vi "Actor Core.vi"(8 "error in":errorcluster, 11 "POLARIS Target Focus Actor in":refnum<class "POLARIS Target Focus Actor.lvclass">) -> (0 "error out":errorcluster, 3 "Actor out":refnum<class "Actor.lvclass">)   [LabVIEW 2014, in "POLARIS Target Focus Actor.lvlib" / "POLARIS Target Focus Actor.lvclass"]
doc: "(<B>Filename</B>: Actor Framework.lvlib:Actor.lvclass:Actor Core.vi)\n\nReceives messages to the actor, reacts to them, and initiates any error handling that may shut the actor down.\n\nDescendant classes may override this VI to append parallel tasks for the actor to complete while it handles messages. Overrides use the Call Parent Method node."
uses:
  POLARIS Target Focus Actor.lvclass
  <vilib>/ActorFramework/Actor/Actor.lvclass
  Utility/Width Method.ctl
  POLARIS TA Focus Display/POLARIS TA Focus Display/POLARIS TA Focus Display.lvclass
  Analyze/Analyze Parameter/Analyze Parameter Energy/Analyze Parameter Energy.lvclass
  Analyze/Analyze Parameter/Analyze Parameter Width Method/Width Method.lvclass
  Analyze/Analyze Parameter/Analyze Parameter Fluence/Analyze Parameter Fluence.lvclass
  Analyze/Analyze Classes/Analyze Q-Factor/Analyze q-Factor.lvclass
  Analyze/Results and Overlays/Results q-Factor/Analyze Results q-Factor.lvclass
  Camera Actors/IMAQdx Actor/IMAQdx Actor/IMAQdx Actor.lvclass
  Display Actors/HIJ Vision Display/HIJ Vision Display/HIJ Vision Display.lvclass/HIJ Vision Display.ctl
  POLARIS Target Focus Actor.lvclass/POLARIS Target Focus Actor.ctl
  Analyze/Analyze Parameter/Analyze Parameter Energy/Analyze Parameter Energy.lvclass/Analyze Parameter Energy.ctl
  Analyze/Results and Overlays/Results q-Factor/Analyze Results q-Factor.lvclass/Analyze Results q-Factor.ctl
  Applications/HIJ Vision Application/HIJ Vision Application/HIJ Vision Application.lvclass/HIJ Vision Application.ctl
  Applications/HIJ Vision Camera App/HIJ Vision Camera App/HIJ Vision Camera App.lvclass/HIJ Vision Camera App.ctl
  Shared Code/Viewable Actor/ViewableActor/ViewableActor.lvclass/ViewableActor.ctl
  <vilib>/ActorFramework/Actor/Actor.lvclass/Actor.ctl
  <vilib>/ActorFramework/Message Enqueuer/Message Enqueuer.lvclass/Message Enqueuer.ctl
  Applications/HIJ Vision Application/HIJ Vision Application Messages/Set Parameter Msg/Set Parameter Msg.lvclass/Set Parameter Msg.ctl
  Analyze/Analyze Parameter/Analyze Parameter Energy/Write Energy.vi
  Analyze/Results and Overlays/Results q-Factor/Write A ref .vi
  Analyze/Results and Overlays/Results q-Factor/Write q ref.vi
  Display Actors/HIJ Vision Display/HIJ Vision Display/Write Save Report_.vi
  Applications/HIJ Vision Application/HIJ Vision Application/Write SubPnl for Display.vi
  Applications/HIJ Vision Camera App/HIJ Vision Camera App/Write Child Menu.vi
  Applications/HIJ Vision Application/HIJ Vision Application/Write HIJ Vision Display.vi
  Applications/HIJ Vision Application/HIJ Vision Application/Write Analyze Objs.vi
  Applications/HIJ Vision Camera App/HIJ Vision Camera App/Write Camera Actor.vi
  Shared Code/Viewable Actor/ViewableActor/Write UI VI Ref.vi
  <vilib>/ActorFramework/Message Enqueuer/Init from Existing Queue.vi
  <vilib>/ActorFramework/Message Enqueuer/Enqueue.vi
  <vilib>/ActorFramework/Message Priority Queue/Priority Enqueue.vi
  <vilib>/ActorFramework/Message Enqueuer/Message Enqueuer.lvclass
  <vilib>/ActorFramework/Stop Msg/Stop Msg.lvclass
  Applications/HIJ Vision Application/HIJ Vision Application Messages/Set Parameter Msg/Set Parameter Msg.lvclass
  Applications/HIJ Vision Camera App/HIJ Vision Camera App/HIJ Vision Camera App.lvclass
  Utility/POLARIS Vision utility.lvlib
panel:
  in  "Stop Signal":bool
  out "q-Factor":dbl format="%#_3g"
  out "A":dbl[unit] format="%#.1g"
  out "I [W/cm^2]":dbl[unit] format="%#.2g"
  in  "Energy":dbl[unit]=10.0
  in  "Size of hot Region":i32=10
  in  "Method":T1
  in  "Pulse duration":dbl[unit]=1e-13
  in  "Compressor eff.":dbl=0.63
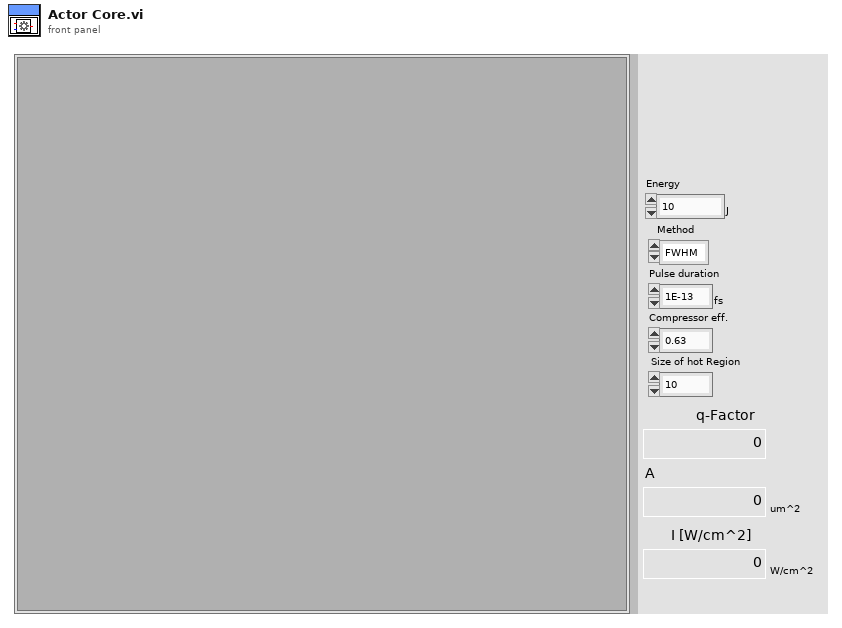
[diagram p1: front panel]
types:
  T1 = typedef "POLARIS Vision utility.lvlib/Width Method.ctl" = enum16{"FWHM", "1/e", "1/e^2", "80%", "90%"}
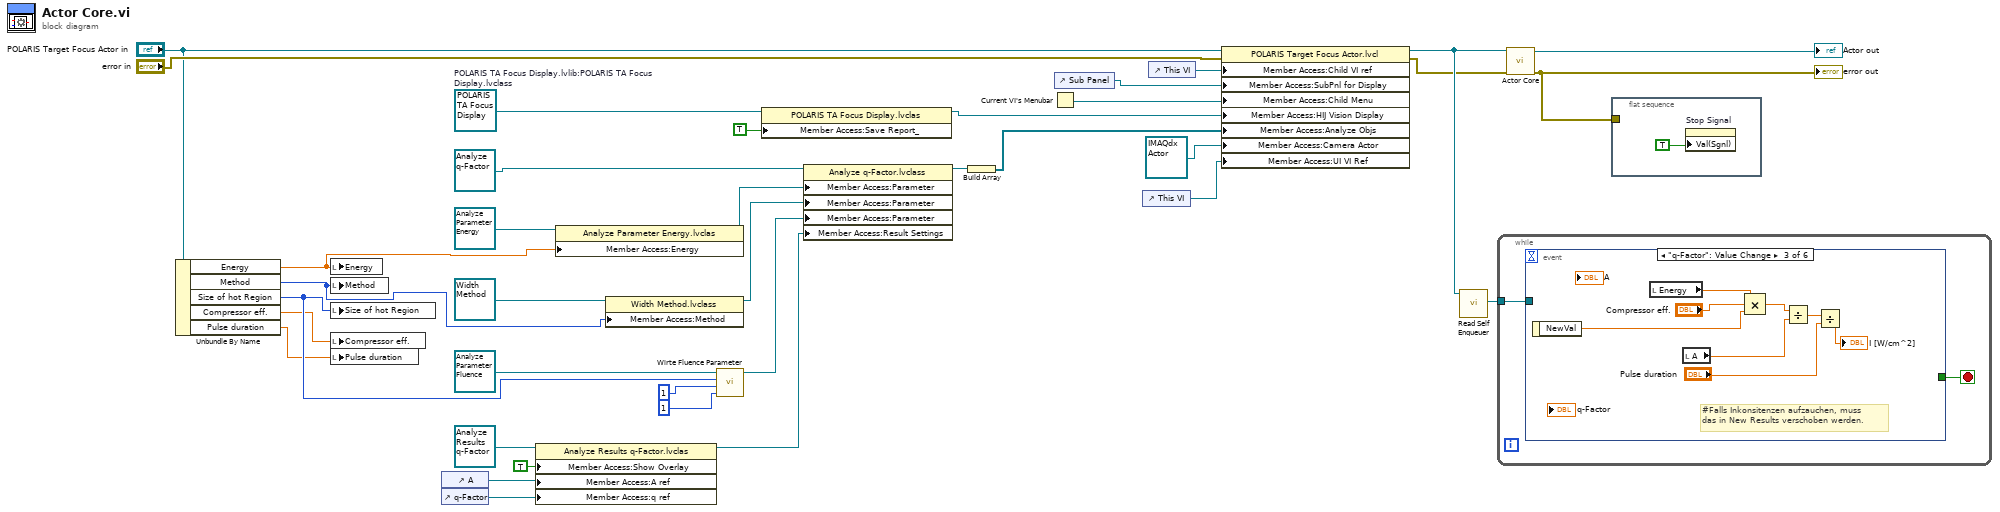
[diagram p0: block diagram]
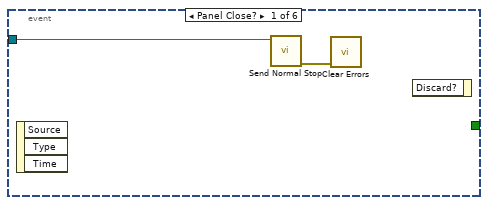
[diagram p2: hidden frame]
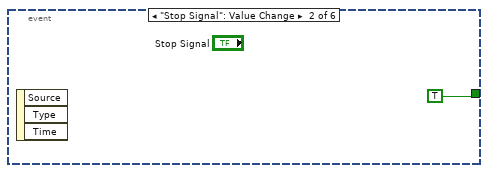
[diagram p3: hidden frame]
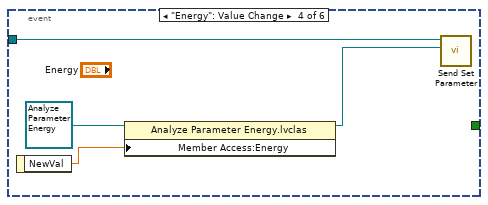
[diagram p4: hidden frame]
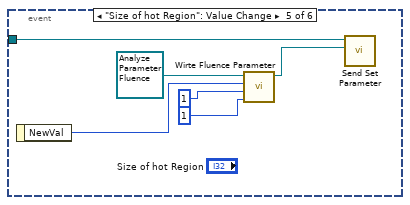
[diagram p5: hidden frame]
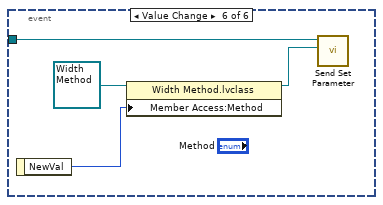
[diagram p6: hidden frame]
diagram:
  w11 = refnum<class "POLARIS TA Focus Display.lvclass"> refnum  # POLARIS TA Focus Display.lvlib:POLARIS TA Focus Display.lvclass
  n1 = Unbundle By Name("POLARIS Target Focus Actor in") -> ("Energy"=w6:dbl[unit], "Method"=w5:T1, "Size of hot Region"=w3:i32, "Compressor eff."=w2:dbl, "Pulse duration"=w1:dbl[unit])
  n2 = local write "Energy"(w6) -> ()
  n3 = local write "Method"(w5) -> ()
  n4 = local write "Size of hot Region"(w3) -> ()
  n5 = local write "Compressor eff."(w2) -> ()
  n6 = local write "Pulse duration"(w1) -> ()
  n7 = control-ref of="A"() -> (w19:refnum<vi>)
  n8 = control-ref of="q-Factor"() -> (w20:refnum<vi>)
  n9 = property class="Analyze Results q-Factor.lvclas"(reference=refnum<class "Analyze Results q-Factor.lvclass"> refnum ("Analyze Results q-Factor.lvclass"), "Member Access:Show Overlay"=TRUE ("Show Overlay"), "Member Access:A ref "=w19, "Member Access:q ref"=w20) -> (reference out=w21:refnum<class "Analyze Results q-Factor.lvclass">)  [unwired: 1 in, 1 out]
  n10 = property class="Analyze Parameter Energy.lvclas"(reference=refnum<class "Analyze Parameter Energy.lvclass"> refnum ("Analyze Parameter Energy.lvclass"), "Member Access:Energy"=w6) -> (reference out=w26:refnum<class "Analyze Parameter Energy.lvclass">)  [unwired: 1 in, 1 out]
  n11 = property class="Width Method.lvclass"(reference=refnum<class "Width Method.lvclass"> refnum ("Width Method.lvclass"), "Member Access:Method"=w5) -> (reference out=w25:refnum<class "Width Method.lvclass">)  [unwired: 1 in, 1 out]
  n12 = call "Wirte Fluence Parameter.vi"("#of Areas"=1, "#Overlays"=1, "Size of region (px)"=w3, "Analyze Parameter Fluence in"=refnum<class "Analyze Parameter Fluence.lvclass"> refnum ("Analyze Parameter Fluence.lvclass")) -> ("Analyze Parameter Fluence out"=w24:refnum<class "Analyze Parameter Fluence.lvclass">)  [unwired: 7 in]
  n13 = property class="POLARIS TA Focus Display.lvclas"(reference=w11, "Member Access:Save Report_"=TRUE ("Save Report_")) -> (reference out=w10:refnum<class "POLARIS TA Focus Display.lvclass">)  [unwired: 1 in, 1 out]
  n14 = property class="Analyze q-Factor.lvclass"(reference=refnum<class "Analyze q-Factor.lvclass"> refnum ("Analyze.lvlib:Analyze q-Factor.lvclass"), "Member Access:Parameter"=w26, "Member Access:Parameter"=w25, "Member Access:Parameter"=w24, "Member Access:Result Settings"=w21) -> (reference out=w14:refnum<class "Analyze q-Factor.lvclass">)  [unwired: 1 in, 1 out]
  n15 = Build Array(w14) -> (w13:refnum<class "Analyze q-Factor.lvclass">[])
  n16 = Current VI's Menubar() -> (w15:refnum<k9>)
  n17 = control-ref of="Sub Panel"() -> (w8:refnum<vi>)
  n18 = control-ref of="This VI"() -> (w16:refnum<vi>)
  n19 = control-ref of="This VI"() -> (w18:refnum<vi>)
  n20 = property class="POLARIS Target Focus Actor.lvcl"(reference="POLARIS Target Focus Actor in", error in="error in", "Member Access:Child VI ref"=w18, "Member Access:SubPnl for Display"=w8, "Member Access:Child Menu"=w15, "Member Access:HIJ Vision Display"=w10, "Member Access:Analyze Objs"=w13, "Member Access:Camera Actor"=refnum<class "IMAQdx Actor.lvclass"> refnum ("IMAQdx Actor.lvlib:IMAQdx Actor.lvclass"), "Member Access:UI VI Ref"=w16) -> (reference out=w36:refnum<class "POLARIS Target Focus Actor.lvclass">, error out=w32:errorcluster)
  n21 = call <vilib>:"Read Self Enqueuer.vi"("Actor"=w36) -> ("Self Enqueuer"=w35:refnum<class "Message Enqueuer.lvclass">)  [unwired: 10 in]
  n22 = while {
    tunnel: w35 -> [w37]
    stop <- w38 stop-if-true
    n23 = event shown="[2] \"q-Factor\": Value Change" {
      selector: _ -> [_ _ _ _ _ _]
      dyn-events: _ -> [_ _ _ _ _ _]
      timeout: _ -> [_ _ _ _ _ _]
      tunnel: [_ TRUE _ _ _ _] -> w38
      tunnel: w37 -> [w40 _ _ w51 w55 w63]
      event Panel Close? {
        n24 = event-data() -> ()  [unwired: 1 in, 3 out]
        n25 = call <vilib>:"Send Normal Stop.vi"("Message Enqueuer"=w40) -> ("error out"=w39:errorcluster)  [unwired: 10 in]
        n26 = call <vilib>:"Clear Errors.vi"("error in (no error)"=w39) -> ()  [unwired: 5 in, 2 out]
        n27 = event-data() -> ()  [unwired: 2 in, 1 out]
      }
      event "Stop Signal": Value Change {
        n28 = event-data() -> ()  [unwired: 1 in, 3 out]
      }
      event "q-Factor": Value Change {
        # "#Falls Inkonsitenzen aufzauchen, muss\ndas in New Results verschoben werden."
        n29 = event-data() -> ("NewVal"=w47:dbl)  [unwired: 1 in]
        n30 = local read "Energy"() -> (w48:dbl[unit])
        n31 = local read "A"() -> (w44:dbl[unit])
        n32 = Compound Arithmetic op=MULTIPLY(w48, "Compressor eff.", w47) -> (w46:dbl[unit])
        n33 = Divide(x=w46, y=w44) -> (x/y=w45:dbl[unit])
        n34 = Divide(x=w45, y="Pulse duration") -> (x/y=→"I [W/cm^2]":dbl[unit])
      }
      event "Energy": Value Change {
        n35 = event-data() -> ("NewVal"=w52:dbl[unit])  [unwired: 1 in]
        n36 = property class="Analyze Parameter Energy.lvclas"(reference=refnum<class "Analyze Parameter Energy.lvclass"> refnum ("Analyze Parameter Energy.lvclass"), "Member Access:Energy"=w52) -> (reference out=w50:refnum<class "Analyze Parameter Energy.lvclass">)  [unwired: 1 in, 1 out]
        n37 = call "Send Set Parameter.vi"("Parameter"=w50, "Message Enqueuer"=w51) -> ()  [unwired: 8 in, 2 out]
      }
      event "Size of hot Region": Value Change {
        n38 = event-data() -> ("NewVal"=w56:i32)  [unwired: 1 in]
        n39 = call "Wirte Fluence Parameter.vi"("#of Areas"=1, "#Overlays"=1, "Size of region (px)"=w56, "Analyze Parameter Fluence in"=refnum<class "Analyze Parameter Fluence.lvclass"> refnum ("Analyze Parameter Fluence.lvclass")) -> ("Analyze Parameter Fluence out"=w54:refnum<class "Analyze Parameter Fluence.lvclass">)  [unwired: 7 in]
        n40 = call "Send Set Parameter.vi"("Parameter"=w54, "Message Enqueuer"=w55) -> ()  [unwired: 8 in, 2 out]
      }
      event Value Change {
        n41 = event-data() -> ("NewVal"=w61:T1)  [unwired: 1 in]
        n42 = property class="Width Method.lvclass"(reference=refnum<class "Width Method.lvclass"> refnum ("Width Method.lvclass"), "Member Access:Method"=w61) -> (reference out=w60:refnum<class "Width Method.lvclass">)  [unwired: 1 in, 1 out]
        n43 = call "Send Set Parameter.vi"("Parameter"=w60, "Message Enqueuer"=w63) -> ()  [unwired: 8 in, 2 out]
      }
    }
  }
  n44 = call-parent "Actor Core.vi"("error in"=w32, "HIJ Vision Camera App In"=w36) -> ("error out"=w33:errorcluster, "Actor out"=→"Actor out":refnum<class "Actor.lvclass">)  [unwired: 8 in]
  "error out" <- w33
  n45 = flat-sequence {
    tunnel: w33 -> [_]
    frame #0 {
      n46 = property on="Stop Signal" class="Bool (strict)"("Val(Sgnl)"=TRUE) -> ()  [unwired: 2 in, 2 out]
    }
  }
